vi "ProFile_Measure_test.vi"(1 "Ceiling":sgl=3.0, 3 "error in":errorcluster caption="Error In") -> (0 "error out":errorcluster caption="Error Out")   [LabVIEW 2016]
doc: "2D motor scan example Vi."
uses:
  Utility/Global Constants.vi
  Utility/Global_Array.vi
  Utility/Global_Stage.vi
panel:
  in  "Y-Axis Scanner align":sgl=0.09
  in  "X-Axis Scanner align":sgl=-0.495
  out "Value Handle":dbl[](array[numeric])
  out "Status?":bool
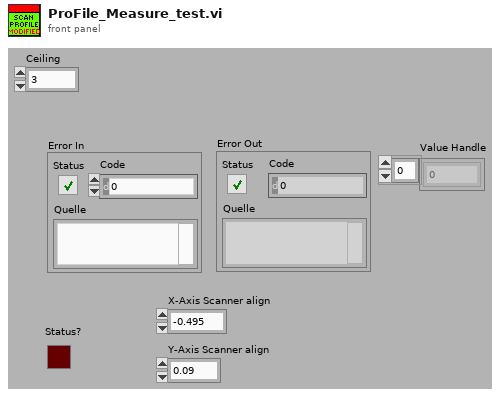
[diagram p1: front panel]
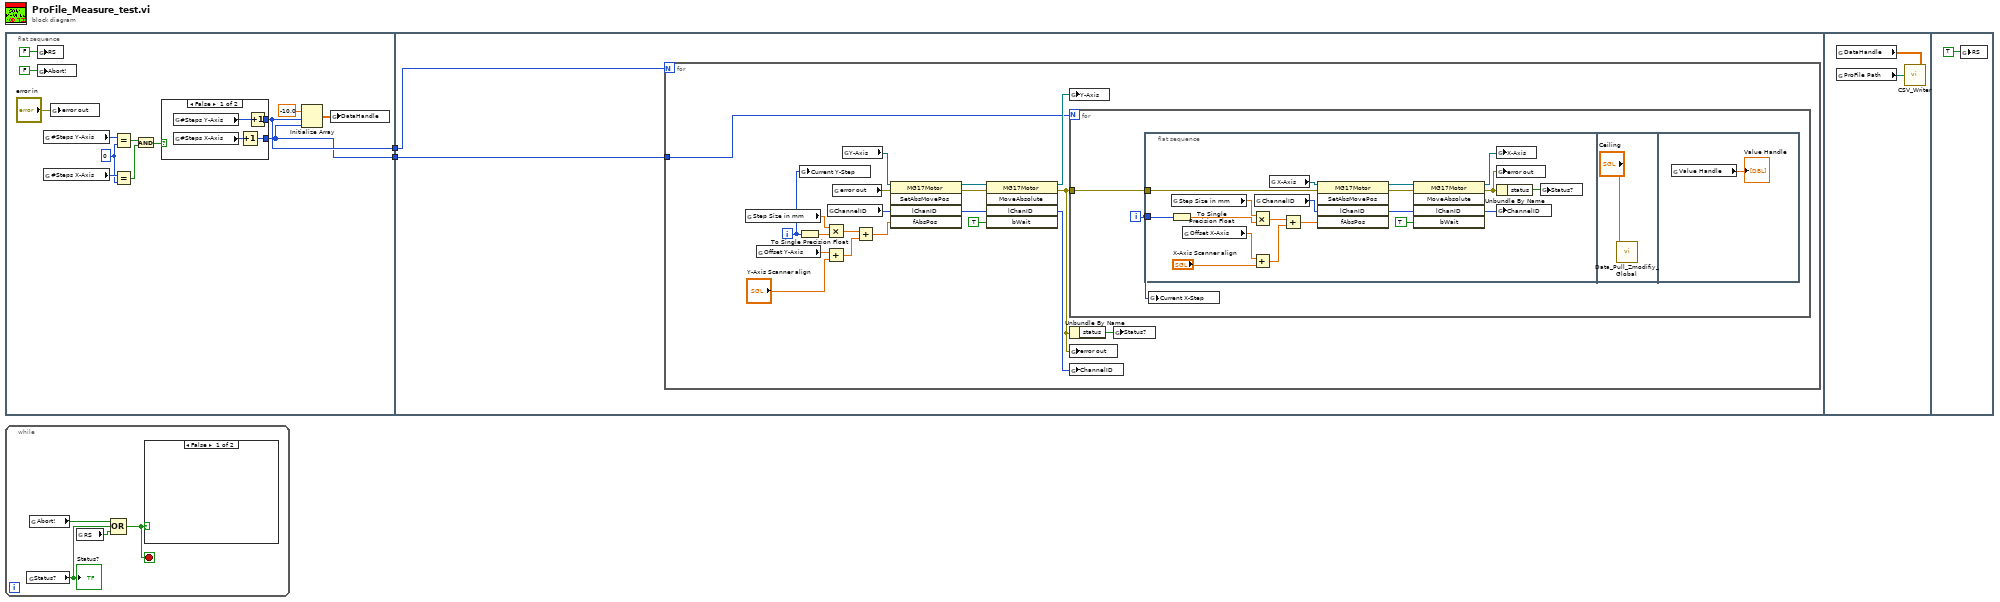
[diagram p0: block diagram]
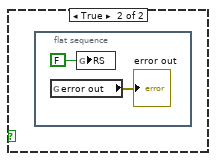
[diagram p2: hidden frame]
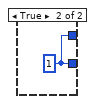
[diagram p3: hidden frame]
diagram:
  n1 = flat-sequence {
    tunnel: [w5] -> w2
    tunnel: [w4] -> w1
    tunnel: w2 -> [w22]
    tunnel: w1 -> [w21]
    frame #0 {
      w7 = 0 ("y")
      n2 = global write "Global Constants.vi" "RS"(FALSE ("Run Successful")) -> ()
      n3 = global write "Global Constants.vi" "Abort!"(FALSE) -> ()
      n4 = global read "Global Constants.vi" "#Steps Y-Axis"() -> (w12:i32)
      n5 = global read "Global Constants.vi" "#Steps X-Axis"() -> (w8:i32)
      n6 = global write "Global Constants.vi" "error out"("error in") -> ()
      n7 = Equal?(x=w12, y=w7) -> (x = y?=w11:bool)
      n8 = Equal?(x=w8, y=w7) -> (x = y?=w10:bool)
      n9 = And(x=w11, y=w10) -> (x .and. y?=w9:bool)
      n10 = case shown="False" w9 {
        tunnel: [w17 w20] -> w5
        tunnel: [w16 w20] -> w4
        frame False {
          n11 = global read "Global Constants.vi" "#Steps Y-Axis"() -> (w19:i32)
          n12 = global read "Global Constants.vi" "#Steps X-Axis"() -> (w18:i32)
          n13 = Increment(x=w18) -> (x+1=w16:i32)
          n14 = Increment(x=w19) -> (x+1=w17:i32)
        }
        frame True {
          w20 = 1
        }
      }
      n15 = Initialize Array(sgl -10.0 ("element"), w5, w4) -> (w15:sgl[][])
      n16 = global write "Global_Array.vi" "DataHandle"(w15) -> ()
    }
    frame #1 {
      n17 = for {
        N: w22 -> [_]
        tunnel: w21 -> [w23]
        i -> [w27]
        n18 = global read "Global Constants.vi" "Step Size in mm"() -> (w34:sgl)
        n19 = global read "Global Constants.vi" "Offset Y-Axis"() -> (w25:sgl)
        n20 = To Single Precision Float(number=w27) -> (single precision float=w39:sgl)
        n21 = global write "Global Constants.vi" "Current Y-Step"(w27) -> ()
        n22 = Multiply(x=w34, y=w39) -> (x*y=w37:sgl)
        n23 = Add(x=w25, y="Y-Axis Scanner align") -> (x+y=w24:sgl)
        n24 = global read "Global_Stage.vi" "ChannelID"() -> (w32:i32)
        n25 = global read "Global Constants.vi" "error out"() -> (w28:errorcluster)
        n26 = global read "Global_Stage.vi" "Y-Axis"() -> (w33:refnum<k7>)
        n27 = Add(x=w37, y=w24) -> (x+y=w36:sgl)
        n28 = invoke class="MG17Motor" method="SetAbsMovePos"(reference=w33, error in=w28, "lChanID"=w32, "fAbsPos"=w36) -> (reference out=w38:refnum<k7>, error out=w42:errorcluster, "lChanID"=w40:i32)  [unwired: 1 in, 2 out]
        n29 = invoke class="MG17Motor" method="MoveAbsolute"(reference=w38, error in=w42, "lChanID"=w40, "bWait"=TRUE) -> (reference out=w30:refnum<k7>, error out=w29:errorcluster, "lChanID"=w31:i32)  [unwired: 1 in, 2 out]
        n30 = global write "Global_Stage.vi" "Y-Axis"(w30) -> ()
        n31 = for {
          N: w23 -> [_]
          tunnel: w29 -> [w44]
          i -> [w43]
          n32 = flat-sequence {
            tunnel: w43 -> [w58]
            tunnel: w44 -> [w48]
            frame #0 {
              n33 = To Single Precision Float(number=w58) -> (single precision float=w60:sgl)
              n34 = global read "Global Constants.vi" "Step Size in mm"() -> (w53:sgl)
              n35 = global read "Global Constants.vi" "Offset X-Axis"() -> (w47:sgl)
              n36 = Multiply(x=w53, y=w60) -> (x*y=w57:sgl)
              n37 = Add(x=w47, y="X-Axis Scanner align") -> (x+y=w45:sgl)
              n38 = global read "Global_Stage.vi" "ChannelID"() -> (w51:i32)
              n39 = global read "Global_Stage.vi" "X-Axis"() -> (w52:refnum<k7>)
              n40 = Add(x=w57, y=w45) -> (x+y=w56:sgl)
              n41 = invoke class="MG17Motor" method="SetAbsMovePos"(reference=w52, error in=w48, "lChanID"=w51, "fAbsPos"=w56) -> (reference out=w59:refnum<k7>, error out=w63:errorcluster, "lChanID"=w62:i32)  [unwired: 1 in, 2 out]
              n42 = invoke class="MG17Motor" method="MoveAbsolute"(reference=w59, error in=w63, "lChanID"=w62, "bWait"=TRUE) -> (reference out=w50:refnum<k7>, error out=w55:errorcluster, "lChanID"=w49:i32)  [unwired: 1 in, 2 out]
              n43 = global write "Global_Stage.vi" "X-Axis"(w50) -> ()
              n44 = global write "Global Constants.vi" "error out"(w55) -> ()
              n45 = Unbundle By Name(w55) -> ("status"=w54:bool)
              n46 = global write "Global_Stage.vi" "ChannelID"(w49) -> ()
              n47 = global write "Global Constants.vi" "Status?"(w54) -> ()
            }
            frame #1 {
              n48 = call "Data_Pull_Zmodifiy_Global.vi"("Ceiling"="Ceiling") -> ()
            }
            frame #2 {
              n49 = global read "Global_Array.vi" "Value Handle"() -> (→"Value Handle":dbl[])
            }
          }
          n50 = global write "Global Constants.vi" "Current X-Step"(w43) -> ()
        }
        n51 = Unbundle By Name(w29) -> ("status"=w35:bool)
        n52 = global write "Global Constants.vi" "error out"(w29) -> ()
        n53 = global write "Global_Stage.vi" "ChannelID"(w31) -> ()
        n54 = global write "Global Constants.vi" "Status?"(w35) -> ()
      }
    }
    frame #2 {
      n55 = global read "Global_Array.vi" "DataHandle"() -> (w67:sgl[][])
      n56 = global read "Global Constants.vi" "ProFile Path"() -> (w66:path)
      n57 = call "CSV_Writer.vi"("Array In"=w67, "ProFile In"=w66) -> ()
    }
    frame #3 {
      n58 = global write "Global Constants.vi" "RS"(TRUE) -> ()
    }
  }
  n59 = while {
    stop <- w72 stop-if-true
    n60 = global read "Global Constants.vi" "Status?"() -> (w71:bool)
    "Status?" <- w71
    n61 = global read "Global Constants.vi" "Abort!"() -> (w70:bool)
    n62 = global read "Global Constants.vi" "RS"() -> (w69:bool)
    n63 = Compound Arithmetic op=OR(w70, w71, w69) -> (w72:bool)
    n64 = case shown="False" w72 {
      frame False {
      }
      frame True {
        n65 = flat-sequence {
          frame #0 {
            n66 = global read "Global Constants.vi" "error out"() -> (→"error out":errorcluster)
            n67 = global write "Global Constants.vi" "RS"(FALSE) -> ()
          }
        }
      }
    }
  }
